vi "Unit Test.vi"() -> ()   [LabVIEW 2018]
uses:
  PPLs/Power Supply/Parent/Power_Supply.lvlibp/Custom Control/Supply Settings.ctl
  2230G.lvclass
  PPLs/Power Supply/Parent/Power_Supply.lvlibp/Power Supply.lvclass
  PPLs/Power Supply/Parent/Power_Supply.lvlibp/Custom Control/Channel List.ctl
  PPLs/Power Supply/Parent/Power_Supply.lvlibp
  C:/Projects/LabVIEW/PPLs/Power Supply/Parent/Power_Supply.lvlibp/Power Supply.lvclass
  <instrlib>/Keithley KE22xx Series/Keithley KE22xx Series.lvlib
panel:
  in  "MAX Voltage Limit":dbl=8.0 format="%#_13g"
  in  "Channel Select":enum16{"Channel 1", "Channel 2", "Channel 3"}(ring)=enum."Channel 2"
  in  "Enable Max. Voltage (T: Enable)":bool
  in  "Query":bool
  in  "Set Protection":bool
  out "Output":bool[](array[boolean])
  in  "CH 3 Settings":T1
  in  "CH 2 Settings":T1
  in  "CH 1 Settings":T1
  in  "stop":bool
  in  "Reset":bool
  in  "Set CH 3":bool
  in  "Set CH 2":bool
  in  "Set CH 1":bool
  in  "Read V-I":bool
  out "I":dbl[](array[numeric])
  out "V":dbl[](array[numeric])
  out "error out":errorcluster
  in  "Resource":refnum<visa-resource-name>
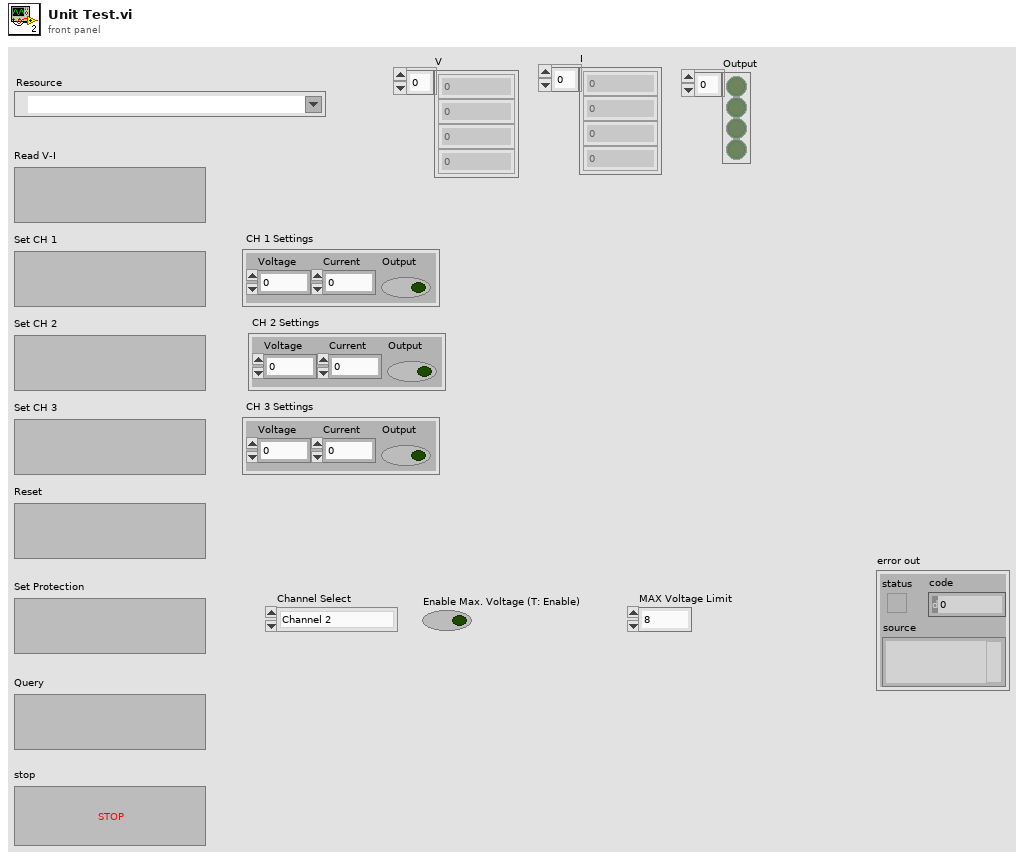
[diagram p1: front panel]
types:
  T1 = typedef "Power_Supply.lvlibp/Supply Settings.ctl" = cluster{"Voltage":dbl, "Current":dbl, "Output":bool}
  T2 = typedef "Power_Supply.lvlibp/Channel List.ctl" = enum16{"Channel 1", "Channel 2", "Channel 3", "Channel 4"}
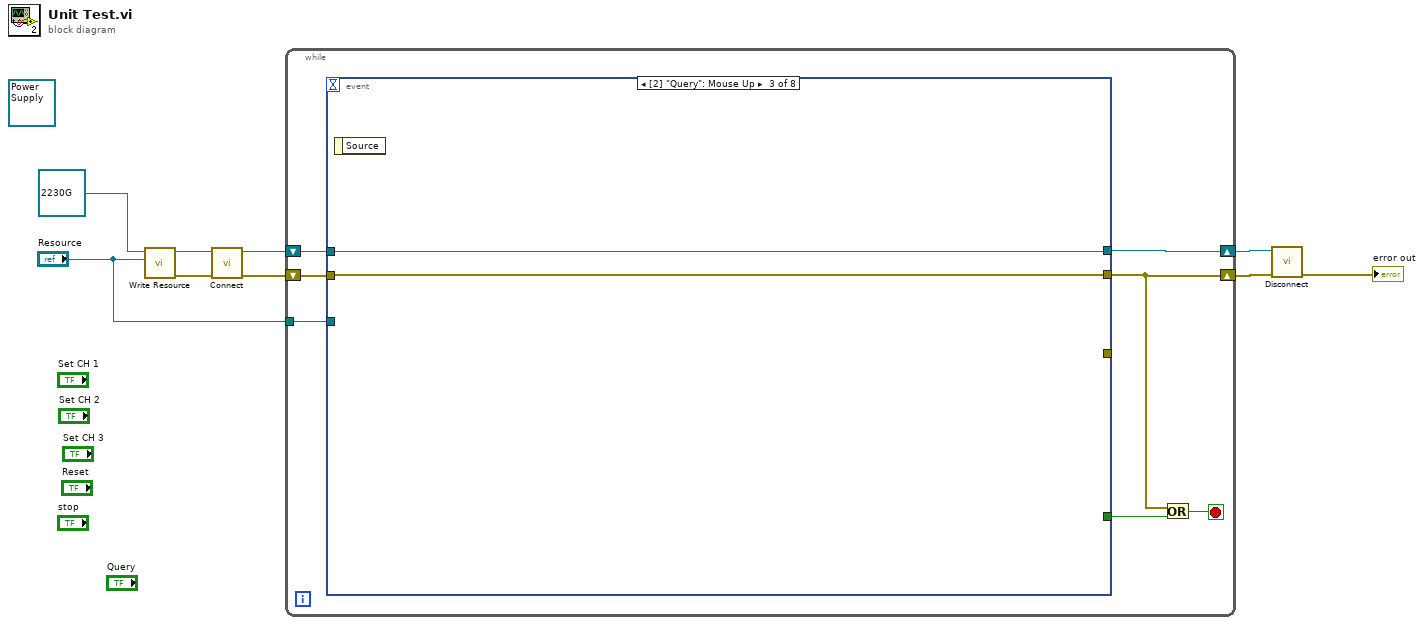
[diagram p0: block diagram]
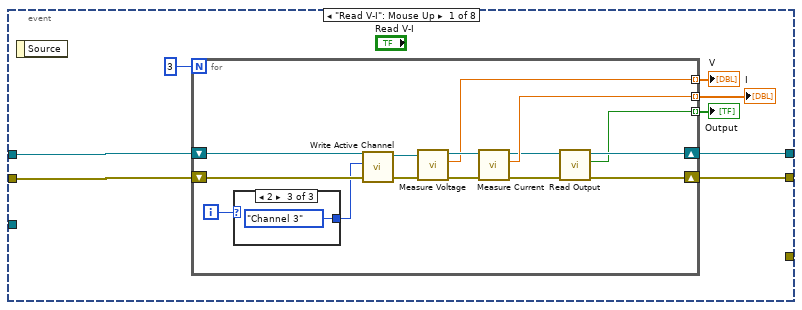
[diagram p2: hidden frame]
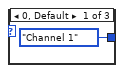
[diagram p3: hidden frame]
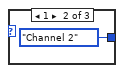
[diagram p4: hidden frame]
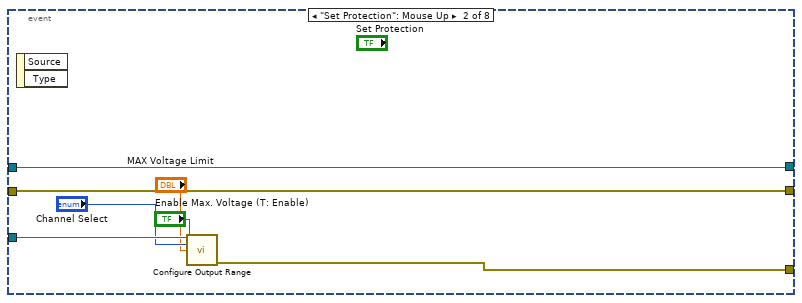
[diagram p5: hidden frame]
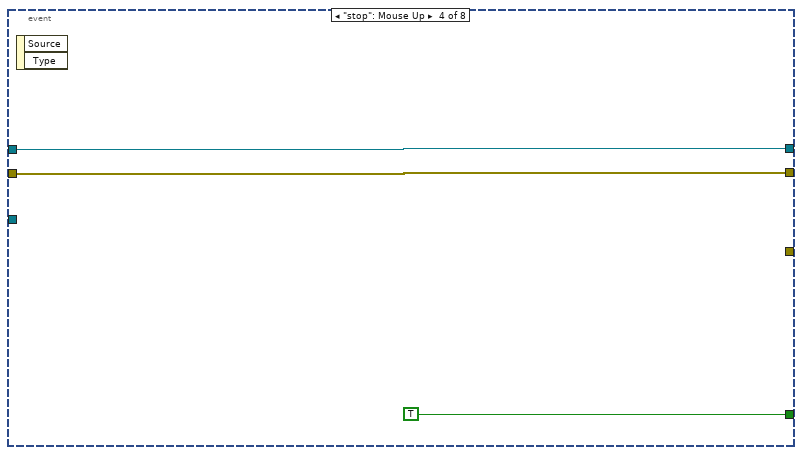
[diagram p6: hidden frame]
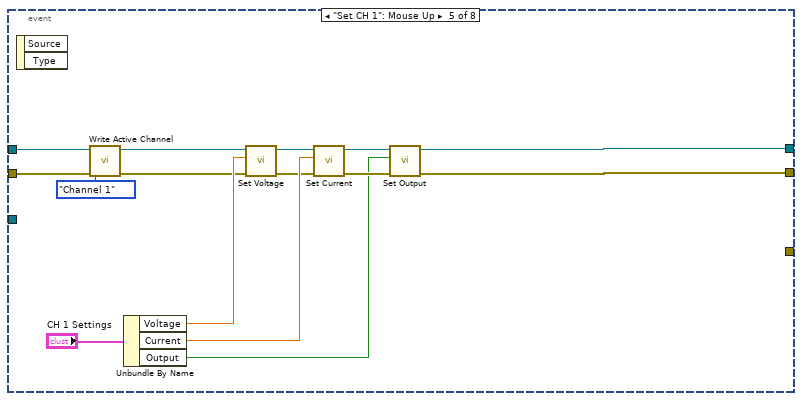
[diagram p7: hidden frame]
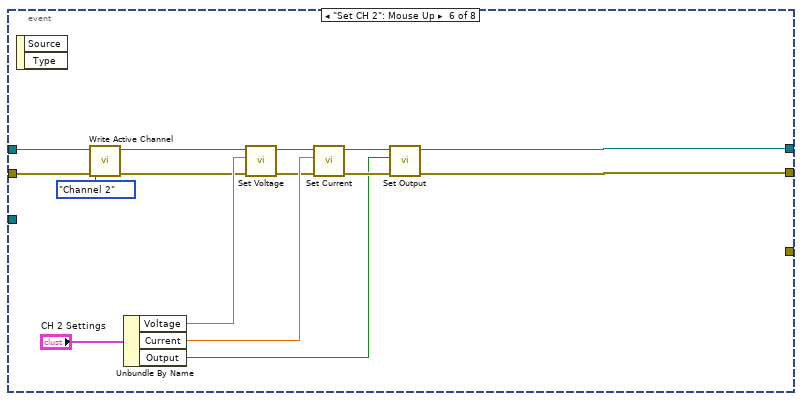
[diagram p8: hidden frame]
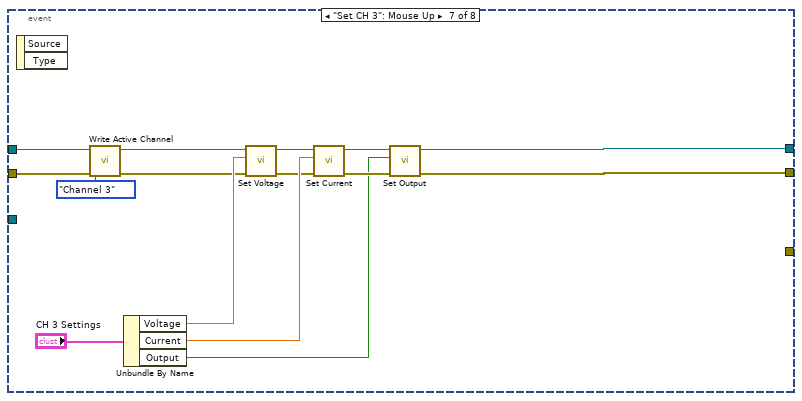
[diagram p9: hidden frame]
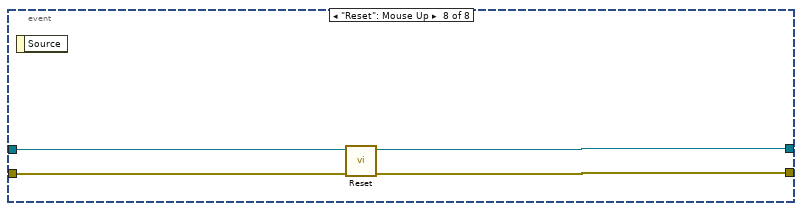
[diagram p10: hidden frame]
diagram:
  (unwired) refnum<class "Power Supply.lvclass"> refnum ("Power_Supply.lvlibp:Power Supply.lvclass")
  n1 = call "Write Resource.vi"("Resource"="Resource", "Power Supply in"=refnum<class "2230G.lvclass"> refnum ("2230G.lvlib:2230G.lvclass")) -> ("error out"=w7:errorcluster, "Power Supply out"=w8:refnum<class "2230G.lvclass">)  [unwired: 8 in]
  n2 = call-dynamic "Connect.vi"("error in (no error)"=w7, "2230G in"=w8) -> ("error out"=w5:errorcluster, "2230G out"=w4:refnum<class "2230G.lvclass">)  [unwired: 8 in]
  n3 = while {
    shift-right: [w12] -> w2
    shift-left: w5 -> [w16]
    shift-right: [w14] -> w3
    shift-left: w4 -> [w15]
    tunnel: "Resource" -> [w10]
    stop <- w13 stop-if-true
    n4 = event shown="[2] \"Query\": Mouse Up" {
      selector: _ -> [_ _ _ _ _ _ _ _]
      dyn-events: _ -> [_ _ _ _ _ _ _ _]
      timeout: _ -> [_ _ _ _ _ _ _ _]
      tunnel: w16 -> [w18 w45 w50 w53 w67 w82 w97 w102]
      tunnel: w15 -> [w24 w46 w51 w54 w68 w83 w98 w103]
      tunnel: [w23 w46 w51 w54 w56 w72 w87 w101] -> w14
      tunnel: [w19 w45 w50 w53 w55 w71 w86 w100] -> w12
      tunnel: [_ _ _ TRUE _ _ _ _] -> w11
      tunnel: w10 -> [_ w49 _ _ _ _ _ _]
      tunnel: [_ w44 _ _ _ _ _ _] -> _
      event "Read V-I": Mouse Up {
        n5 = event-data() -> ()  [unwired: 1 in, 1 out]
        n6 = for {
          N: 3 -> [_]
          shift-right: [w26] -> w19
          shift-left: w18 -> [w38]
          tunnel: [w31] -> w21 mode=indexing
          tunnel: [w30] -> w20 mode=indexing
          shift-right: [w27] -> w23
          shift-left: w24 -> [w39]
          tunnel: [w25] -> w17 mode=indexing
          i -> [w36]
          n7 = case shown="2" w36 {
            tunnel: [Channel_List."Channel 1" ("Active Channel") Channel_List."Channel 2" ("Active Channel") Channel_List."Channel 3" ("Active Channel")] -> w37
            frame 0, Default {
            }
            frame 1 {
            }
            frame 2 {
            }
          }
          n8 = call "Write Active Channel.vi"("error in"=w38, "Active Channel"=w37, "Power Supply in"=w39) -> ("error out"=w34:errorcluster, "Power Supply out"=w35:refnum<class "2230G.lvclass">)  [unwired: 7 in]
          n9 = call-dynamic "Measure Voltage.vi"("error in (no error)"=w34, "2230G in"=w35) -> ("error out"=w32:errorcluster, "Voltage"=w31:dbl, "2230G out"=w33:refnum<class "2230G.lvclass">)  [unwired: 7 in]
          n10 = call-dynamic "Measure Current.vi"("error in (no error)"=w32, "2230G in"=w33) -> ("error out"=w28:errorcluster, "Current"=w30:dbl, "2230G out"=w29:refnum<class "2230G.lvclass">)  [unwired: 7 in]
          n11 = call-dynamic "Read Output.vi"("error in"=w28, "2230G in"=w29) -> ("error out"=w26:errorcluster, "Output"=w25:bool, "2230G out"=w27:refnum<class "2230G.lvclass">)  [unwired: 7 in]
        }
        "V" <- w21
        "I" <- w20
        "Output" <- w17
      }
      event "Set Protection": Mouse Up {
        n12 = event-data() -> ()  [unwired: 1 in, 2 out]
        n13 = call <instrlib>:"Configure Output Range.vi"("VISA resource name"=w49, "Channel Select"="Channel Select", "MAX Voltage Limit"="MAX Voltage Limit", "Enable Max. Voltage (T: Enable)"="Enable Max. Voltage (T: Enable)") -> ("error out"=w44:errorcluster)  [unwired: 10 in, 1 out]
      }
      event "Query": Mouse Up {
        n14 = event-data() -> ()  [unwired: 1 in, 1 out]
      }
      event "stop": Mouse Up {
        n15 = event-data() -> ()  [unwired: 1 in, 2 out]
      }
      event "Set CH 1": Mouse Up {
        n16 = event-data() -> ()  [unwired: 1 in, 2 out]
        n17 = call "Write Active Channel.vi"("error in"=w67, "Active Channel"=Channel_List."Channel 1", "Power Supply in"=w68) -> ("error out"=w63:errorcluster, "Power Supply out"=w66:refnum<class "2230G.lvclass">)  [unwired: 7 in]
        n18 = Unbundle By Name("CH 1 Settings") -> ("Voltage"=w64:dbl, "Current"=w61:dbl, "Output"=w57:bool)
        n19 = call "Set Voltage.vi"("error in"=w63, "Voltage"=w64, "Power Supply in"=w66) -> ("error out"=w60:errorcluster, "Power Supply out"=w62:refnum<class "2230G.lvclass">)  [unwired: 7 in]
        n20 = call "Set Current.vi"("error in"=w60, "Current"=w61, "Power Supply in"=w62) -> ("error out"=w58:errorcluster, "Power Supply out"=w59:refnum<class "2230G.lvclass">)  [unwired: 7 in]
        n21 = call "Set Output.vi"("error in"=w58, "Output"=w57, "Power Supply in"=w59) -> ("error out"=w55:errorcluster, "Power Supply out"=w56:refnum<class "2230G.lvclass">)  [unwired: 7 in]
      }
      event "Set CH 2": Mouse Up {
        n22 = event-data() -> ()  [unwired: 1 in, 2 out]
        n23 = call "Write Active Channel.vi"("error in"=w82, "Active Channel"=Channel_List."Channel 2", "Power Supply in"=w83) -> ("error out"=w79:errorcluster, "Power Supply out"=w81:refnum<class "2230G.lvclass">)  [unwired: 7 in]
        n24 = Unbundle By Name("CH 2 Settings") -> ("Voltage"=w80:dbl, "Current"=w77:dbl, "Output"=w73:bool)
        n25 = call "Set Voltage.vi"("error in"=w79, "Voltage"=w80, "Power Supply in"=w81) -> ("error out"=w76:errorcluster, "Power Supply out"=w78:refnum<class "2230G.lvclass">)  [unwired: 7 in]
        n26 = call "Set Current.vi"("error in"=w76, "Current"=w77, "Power Supply in"=w78) -> ("error out"=w74:errorcluster, "Power Supply out"=w75:refnum<class "2230G.lvclass">)  [unwired: 7 in]
        n27 = call "Set Output.vi"("error in"=w74, "Output"=w73, "Power Supply in"=w75) -> ("error out"=w71:errorcluster, "Power Supply out"=w72:refnum<class "2230G.lvclass">)  [unwired: 7 in]
      }
      event "Set CH 3": Mouse Up {
        n28 = event-data() -> ()  [unwired: 1 in, 2 out]
        n29 = call "Write Active Channel.vi"("error in"=w97, "Active Channel"=Channel_List."Channel 3", "Power Supply in"=w98) -> ("error out"=w94:errorcluster, "Power Supply out"=w96:refnum<class "2230G.lvclass">)  [unwired: 7 in]
        n30 = Unbundle By Name("CH 3 Settings") -> ("Voltage"=w95:dbl, "Current"=w92:dbl, "Output"=w88:bool)
        n31 = call "Set Voltage.vi"("error in"=w94, "Voltage"=w95, "Power Supply in"=w96) -> ("error out"=w91:errorcluster, "Power Supply out"=w93:refnum<class "2230G.lvclass">)  [unwired: 7 in]
        n32 = call "Set Current.vi"("error in"=w91, "Current"=w92, "Power Supply in"=w93) -> ("error out"=w89:errorcluster, "Power Supply out"=w90:refnum<class "2230G.lvclass">)  [unwired: 7 in]
        n33 = call "Set Output.vi"("error in"=w89, "Output"=w88, "Power Supply in"=w90) -> ("error out"=w86:errorcluster, "Power Supply out"=w87:refnum<class "2230G.lvclass">)  [unwired: 7 in]
      }
      event "Reset": Mouse Up {
        n34 = event-data() -> ()  [unwired: 1 in, 1 out]
        n35 = call-dynamic "Reset.vi"("error in (no error)"=w102, "2230G in"=w103) -> ("error out"=w100:errorcluster, "2230G out"=w101:refnum<class "2230G.lvclass">)  [unwired: 8 in]
      }
    }
    n36 = Or(x=w12, y=w11) -> (x .or. y?=w13:bool)
  }
  n37 = call-dynamic "Disconnect.vi"("error in (no error)"=w2, "2230G in"=w3) -> ("error out"=→"error out":errorcluster)  [unwired: 8 in, 1 out]
